vi "_API_BINANCE_GET_Depth.vi"(0 "BinanceAPI in":refnum<class "BinanceAPI_.lvclass">, 5 "Depth":T2, 11 "error in (no error)":errorcluster) -> (4 "BinanceAPI out":refnum<class "BinanceAPI_.lvclass">, 6 "data":T1, 14 "Data":string, 15 "error out":errorcluster)   [LabVIEW 2022 SP3, in "BinanceAPI_.lvclass"]
doc: "https://binance-docs.github.io/apidocs/spot/en/#order-books"
uses:
  BinanceAPI_.lvclass
  BinanceAPI_.lvclass/BinanceAPI_.ctl
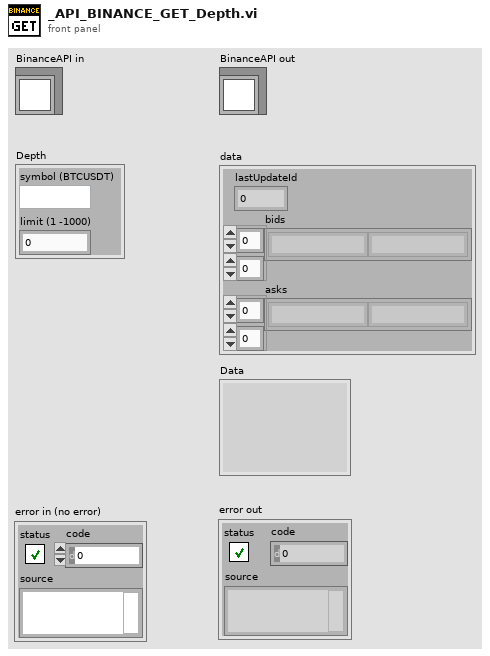
[diagram p1: front panel]
types:
  T1 = cluster{"lastUpdateId":u32, "bids":string[][], "asks":string[][]}
  T2 = cluster{"symbol (BTCUSDT)":string, "limit (1 -1000)":i16}
  T3 = cluster{"lastUpdateId":dbl, "bids":string[][], "asks":string[][]}
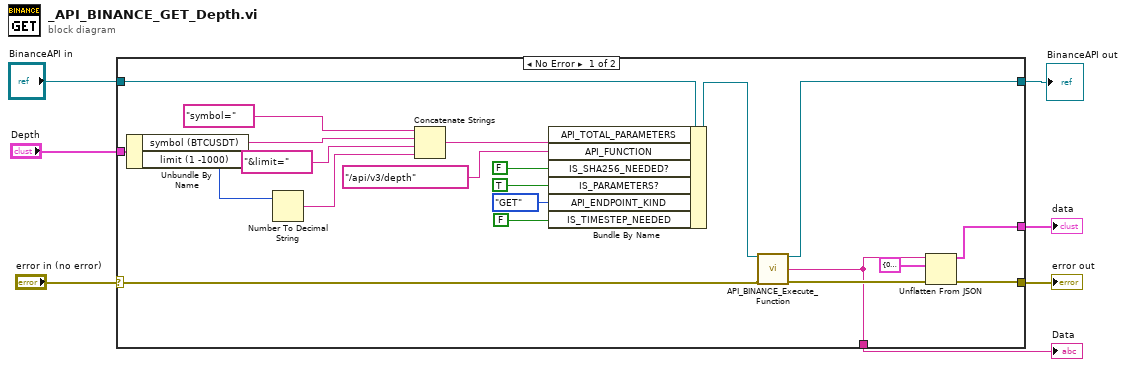
[diagram p0: block diagram]
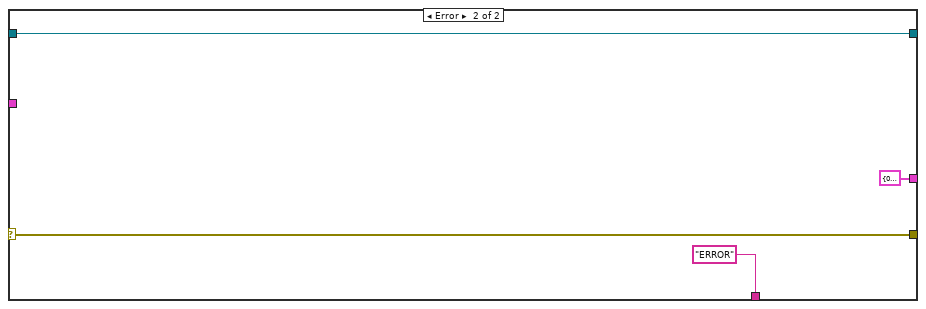
[diagram p2: hidden frame]
diagram:
  n1 = case shown="No Error" "error in (no error)" {
    selector: "error in (no error)" -> [w17 w32]
    tunnel: [w11 w32] -> w5
    tunnel: [w19 w31] -> w2
    tunnel: "BinanceAPI in" -> [w18 w31]
    tunnel: "Depth" -> [w22 _]
    tunnel: [w10 "ERROR" ("Dane")] -> w4
    tunnel: [w8 T1 {"lastUpdateId"=0, "bids"=[], "asks"=[]} ("type and defaults")] -> w3
    frame No Error {
      n2 = Unbundle By Name(w22) -> ("symbol (BTCUSDT)"=w21:string, "limit (1 -1000)"=w15:i16)
      n3 = Number To Decimal String(number=w15) -> (decimal integer string=w14:string)  [unwired: 1 in]
      n4 = Concatenate Strings("symbol=", w21, "&limit=", w14) -> (w23:string)
      n5 = Bundle By Name(cluster=w18, "API_TOTAL_PARAMETERS"=w23, "API_FUNCTION"="/api/v3/depth", "IS_SHA256_NEEDED?"=FALSE, "IS_PARAMETERS?"=TRUE, "API_ENDPOINT_KIND"=enum16{"POST", "DELETE", "GET", "PUT"}."GET", "IS_TIMESTEP_NEEDED"=FALSE) -> (w13:refnum<class "BinanceAPI_.lvclass">)
      n6 = call "API_BINANCE_Execute_Function.vi"("BinanceAPI in"=w13, "error in (no error)"=w17) -> ("BinanceAPI out"=w19:refnum<class "BinanceAPI_.lvclass">, "Body"=w10:string, "error out"=w12:errorcluster)  [unwired: 9 in, 2 out]
      n7 = Unflatten From JSON(JSON string=w10, type and defaults=T3 {"lastUpdateId"=0.0, "bids"=[], "asks"=[]}, error in (no error)=w12) -> (value=w8:T3, error out=w11:errorcluster)  [unwired: 4 in]
    }
    frame Error {
    }
  }
  "error out" <- w5
  "Data" <- w4
  "data" <- w3
  "BinanceAPI out" <- w2
